vi "Detect line orientation.vi"(11 "Coordinates":i32[](array[numeric])) -> (3 "Vertical or Horisontal?":enum16{"Horizontal", "Vertical"}(ring))   [LabVIEW 2013]
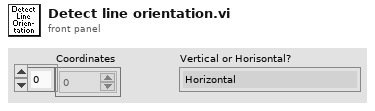
[diagram p1: front panel]
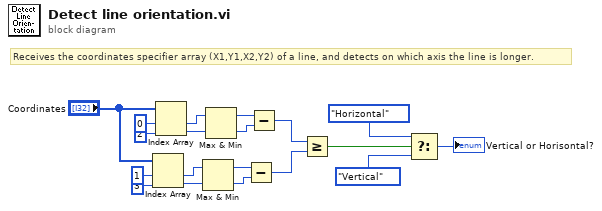
[diagram p0: block diagram]
diagram:
  # "Receives the coordinates specifier array (X1,Y1,X2,Y2) of a line, and detects on which axis the line is longer."
  n1 = Index Array(array="Coordinates", index #1=1 ("index"), index #2=3 ("index")) -> (element #1=w3:i32, element #2=w4:i32)
  n2 = Index Array(array="Coordinates", index #1=0 ("index"), index #2=2 ("index")) -> (element #1=w9:i32, element #2=w10:i32)
  n3 = Max & Min(x=w3, y=w4) -> (max(x,y)=w5:i32, min(x,y)=w6:i32)
  n4 = Max & Min(x=w9, y=w10) -> (max(x,y)=w11:i32, min(x,y)=w12:i32)
  n5 = Subtract(x=w5, y=w6) -> (x-y=w15:i32)
  n6 = Subtract(x=w11, y=w12) -> (x-y=w14:i32)
  n7 = Greater Or Equal?(x=w14, y=w15) -> (x >= y?=w16:bool)
  n8 = Select(t=enum16{"Horizontal", "Vertical"}."Horizontal" ("Line draw mode"), s=w16, f=enum16{"Horizontal", "Vertical"}."Vertical" ("Line draw mode")) -> (s? t:f=→"Vertical or Horisontal?":enum16{"Horizontal", "Vertical"})
